vi "Constructor.vi"(11 "Sample Rate":i32) -> (3 "Mean Fit out":refnum<class "Mean Fit.lvclass">)   [LabVIEW 2016, in "Mean Fit.lvclass"]
uses:
  Mean Fit.lvclass
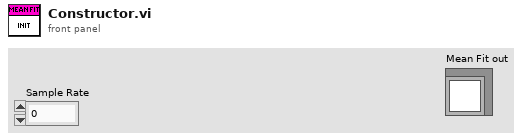
[diagram p1: front panel]
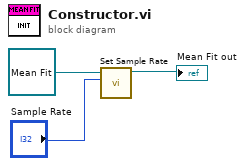
[diagram p0: block diagram]
diagram:
  n1 = call-dynamic "Set Sample Rate.vi"("Sample Rate"="Sample Rate", "Abstract Fit in"=refnum<class "Mean Fit.lvclass"> refnum ("Mean Fit.lvclass")) -> ("Abstract Fit out"=→"Mean Fit out":refnum<class "Mean Fit.lvclass">)  [unwired: 8 in, 1 out]
